vi "Initialize.vi"(8 "error in (no error)":errorcluster, 10 "local path":path) -> (0 "error out":errorcluster, 3 "File Upload Controller out":refnum<class "File Upload Controller.lvclass">)   [LabVIEW 2020, in "NI_SFTP.lvlib" / "File Upload Controller.lvclass"]
uses:
  <vilib>/net/SFTP/API/Support/Upload/File/File Upload Controller.lvclass
  <vilib>/net/SFTP/API/Support/Upload/File/File Upload Controller.lvclass/File Upload Controller.ctl
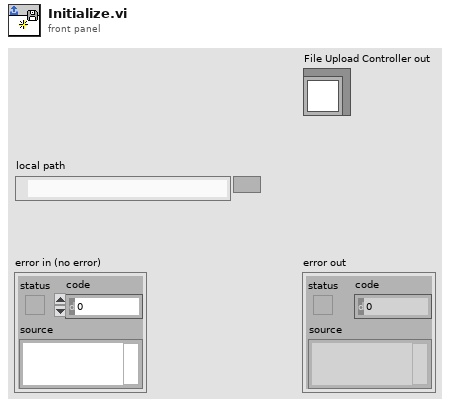
[diagram p1: front panel]
types:
  T1 = enum16{"open", "replace", "create", "open or create", "replace or create", "replace or create with confirmation"}
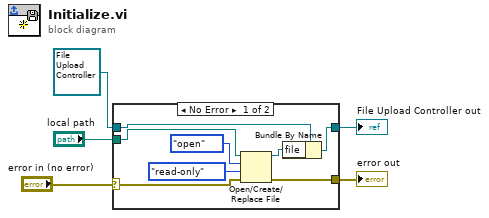
[diagram p0: block diagram]
diagram:
  n1 = case shown="No Error" "error in (no error)" {
    selector: "error in (no error)" -> [w9 w15]
    tunnel: [w8 w15] -> w3
    tunnel: [w7 w14] -> w2
    tunnel: refnum<class "File Upload Controller.lvclass"> refnum ("File Upload Controller in") -> [w6 w14]
    tunnel: "local path" -> [w11 _]
    frame No Error {
      n2 = Open/Create/Replace File(file path (use dialog)=w11, error in=w9, operation (0:open)=T1."open", access (0:read/write)=enum16{"read/write", "read-only", "write-only"}."read-only") -> (refnum out=w10:refnum<file>, error out=w8:errorcluster)  [unwired: 2 in, 1 out]
      n3 = Bundle By Name(cluster=w6, "file"=w10) -> (w7:refnum<class "File Upload Controller.lvclass">)
    }
    frame Error {
    }
  }
  "error out" <- w3
  "File Upload Controller out" <- w2
